vi "LaunchTextLogger.vi"(7 "BufferedLogsInMemory":i32=100, 8 "error in (no error)":errorcluster, 9 "Include Timestamps":bool=TRUE, 10 "Text Log Folder":path, 11 "Parent Actor In (Unwired if root actor)":refnum<class "Actor.lvclass">) -> (0 "error out":errorcluster, 2 "Text Logger Actor's Enqueuer":refnum<class "Message Enqueuer.lvclass">, 3 "Parent Actor Out":refnum<class "Actor.lvclass">)   [LabVIEW 2014, in "EventLogger_Actor.lvlib" / "EventLogger_Actor.lvclass"]
uses:
  EventLogger_Actor.lvclass
  <vilib>/ActorFramework/Actor/Actor.lvclass
  <vilib>/ActorFramework/Message Enqueuer/Message Enqueuer.lvclass
  EventLogger_Actor.lvclass/EventLogger_Actor.ctl
  EventLogger_Actor Messages/CreateBufferQ Msg/CreateBufferQ Msg.lvclass/CreateBufferQ Msg.ctl
  <vilib>/ActorFramework/Message Enqueuer/Message Enqueuer.lvclass/Message Enqueuer.ctl
  <vilib>/ActorFramework/Message Enqueuer/Enqueue.vi
  <userlib>/_OpenG.lib/file/file.llb/Build Path - Traditional__ogtk.vi
  <vilib>/ActorFramework/Message Priority Queue/Priority Enqueue.vi
  EventLogger_Actor Messages/CreateBufferQ Msg/CreateBufferQ Msg.lvclass
  EventLogger_Actor Messages/CreateEventFile Msg/CreateEventFile Msg.lvclass
  EventLogger_Actor.lvlib
panel:
  # "BSD 2-Clause License\n\nCopyright (c) 2018, Ajay www.digiajay.com\nAll rights reserved.\n\nRedistribution and use in source and binary forms, with or without\nmodification, are permitted provided that the following conditions are met:\n\n* Redistributions of source code must retain the above copyright notice, this\n  list of conditions and the following disclaimer.\n\n* Redistributions in binary form must reproduce the above copyright notice,\n  this list of conditions and the following disclaimer in the documentation\n  and/or other materials provided with the distribution.\n\nTHIS SOFTWARE IS PROVIDED BY THE COPYRIGHT HOLDERS AND CONTRIBUTORS \"AS IS\"\nAND ANY EXPRESS OR IMPLIED WARRANTIES, INCLUDING, BUT NOT LIMITED TO, THE\nIMPLIED WARRANTIES OF MERCHANTABILITY AND FITNESS FOR A PARTICULAR PURPOSE ARE\nDISCLAIMED. IN NO EVENT SHALL THE COPYRIGHT HOLDER OR CONTRIBUTORS BE LIABLE\nFOR ANY DIRECT, INDIRECT, INCIDENTAL, SPECIAL, EXEMPLARY, OR CONSEQUENTIAL\nDAMAGES (INCLUDING, BUT NOT LIMITED TO, PROCUREMENT OF SUBSTITUTE GOODS OR\nSERVICES; LOSS OF USE, DATA, OR PROFITS; OR BUSINESS INTERRUPTION) HOWEVER\nCAUSED AND ON ANY THEORY OF LIABILITY, WHETHER IN CONTRACT, STRICT LIABILITY,\nOR TORT (INCLUDING NEGLIGENCE OR OTHERWISE) ARISING IN ANY WAY OUT OF THE USE\nOF THIS SOFTWARE, EVEN IF ADVISED OF THE POSSIBILITY OF SUCH DAMAGE."
  # "Connector Pane"
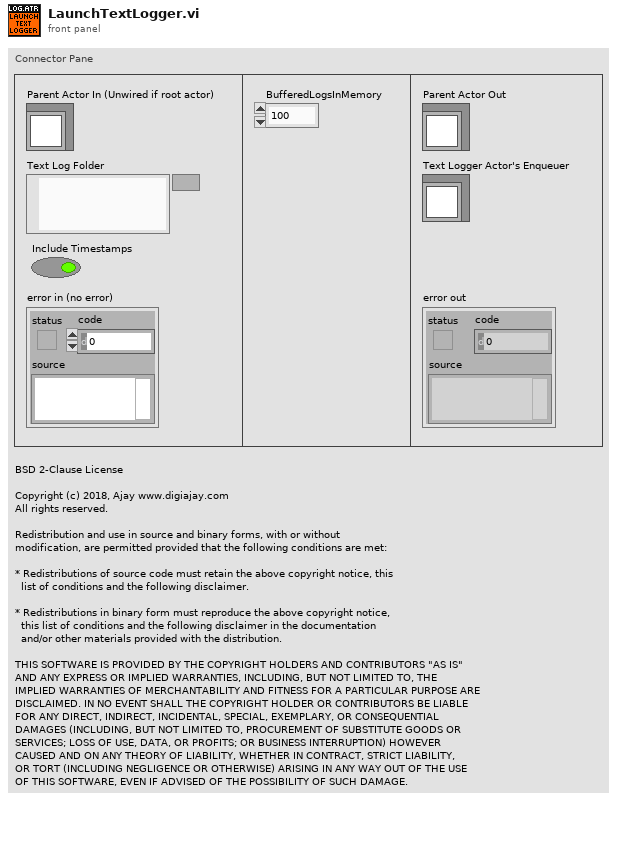
[diagram p1: front panel]
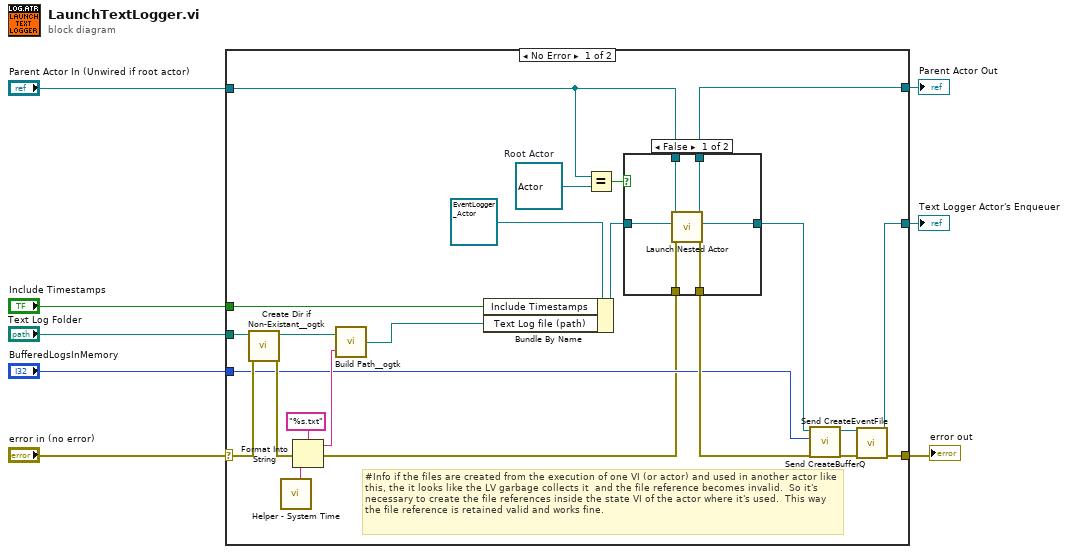
[diagram p0: block diagram]
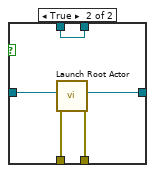
[diagram p2: hidden frame]
diagram:
  n1 = case shown="No Error" "error in (no error)" {
    selector: "error in (no error)" -> [w27 w44]
    tunnel: [w17 w44] -> w7
    tunnel: "Text Log Folder" -> [w26 _]
    tunnel: [w16 _] -> w5
    tunnel: "Parent Actor In (Unwired if root actor)" -> [w18 w43]
    tunnel: [w19 w43] -> w3
    tunnel: "Include Timestamps" -> [w15 _]
    tunnel: "BufferedLogsInMemory" -> [w11 _]
    frame No Error {
      w21 = refnum<class "Actor.lvclass"> refnum  # Root Actor
      # "#Info if the files are created from the execution of one VI (or actor) and used in another actor like this, the it looks like the LV garbage collects it  and the file reference becomes invalid.  So it's necessary to create the file references inside the state VI of the actor where it's used.  This way the file reference is retained valid and works fine."
      n2 = call <userlib>:"Create Dir if Non-Existant__ogtk.vi"("error in (no error)"=w27, "Directory Path"=w26) -> ("error out"=w28:errorcluster, "dup Directory Path"=w25:path)  [unwired: 7 in, 1 out]
      n3 = call "Helper - System Time.vi"() -> ("Date & Time (WinFileFormat)"=w31:string)  [unwired: 7 in, 4 out]
      n4 = Format Into String(format string="%s.txt", error in=w28, w31) -> (resulting string=w29:string, error out=w10:errorcluster)  [unwired: 1 in]
      n5 = call-poly <userlib>:"Build Path__ogtk.vi"("name or relative path"=w29, "base path"=w25) -> ("appended path"=w24:path)
      n6 = Bundle By Name(cluster=refnum<class "EventLogger_Actor.lvclass"> refnum ("object in"), "Include Timestamps"=w15, "Text Log file (path)"=w24) -> (w20:refnum<class "EventLogger_Actor.lvclass">)
      n7 = Equal?(x=w18, y=w21) -> (x = y?=w22:bool)
      n8 = case shown="False" w22 {
        tunnel: w10 -> [w37 w40]
        tunnel: [w36 w41] -> w13
        tunnel: [w35 w38] -> w19
        tunnel: [w34 w39] -> w12
        tunnel: w20 -> [w33 w42]
        tunnel: w18 -> [w32 w38]
        frame False {
          n9 = call <vilib>:"Launch Nested Actor.vi"("error in (no error)"=w37, "Nested Actor"=w33, "Caller Actor in"=w32) -> ("error out"=w36:errorcluster, "Nested Actor's Enqueuer"=w34:refnum<class "Message Enqueuer.lvclass">, "Caller Actor out"=w35:refnum<class "Actor.lvclass">)  [unwired: 6 in]
        }
        frame True {
          n10 = call <vilib>:"Launch Root Actor.vi"("error in (no error)"=w40, "Actor"=w42) -> ("error out"=w41:errorcluster, "Actor's Enqueuer"=w39:refnum<class "Message Enqueuer.lvclass">)  [unwired: 8 in]
        }
      }
      n11 = call "Send CreateBufferQ.vi"("error in (no error)"=w13, "BufferedLogsInMemory"=w11, "Message Enqueuer"=w12) -> ("error out"=w14:errorcluster, "Message Enqueuer out"=w9:refnum<class "Message Enqueuer.lvclass">)  [unwired: 7 in]
      n12 = call "Send CreateEventFile.vi"("error in (no error)"=w14, "Message Enqueuer"=w9) -> ("error out"=w17:errorcluster, "Message Enqueuer out"=w16:refnum<class "Message Enqueuer.lvclass">)  [unwired: 8 in]
    }
    frame Error {
    }
  }
  "error out" <- w7
  "Text Logger Actor's Enqueuer" <- w5
  "Parent Actor Out" <- w3
